vi "rqcBob KeyNET Send Data U32.vi"(8 "error in":errorcluster, 10 "Data":u32[](array[numeric]), 11 "rqcBob KeyNET in":T1) -> (0 "error out":errorcluster, 3 "rqcBob KeyNET out":T1)   [LabVIEW 2016]
uses:
  Custom Controls/rqcBob KeyNET control.ctl
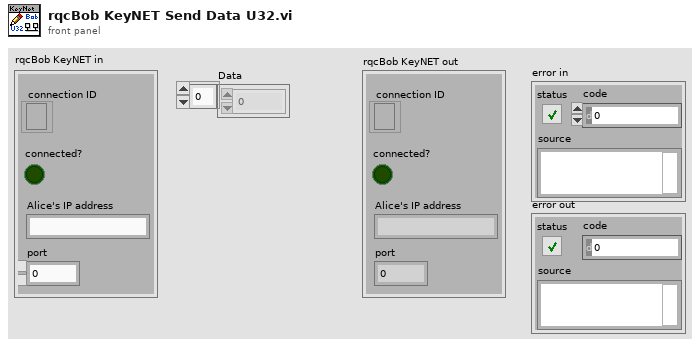
[diagram p1: front panel]
types:
  T1 = typedef "rqcBob KeyNET control.ctl" = cluster{"connection ID":refnum<k5>, "connected?":bool, "Alice's IP address":string, "port":u16}
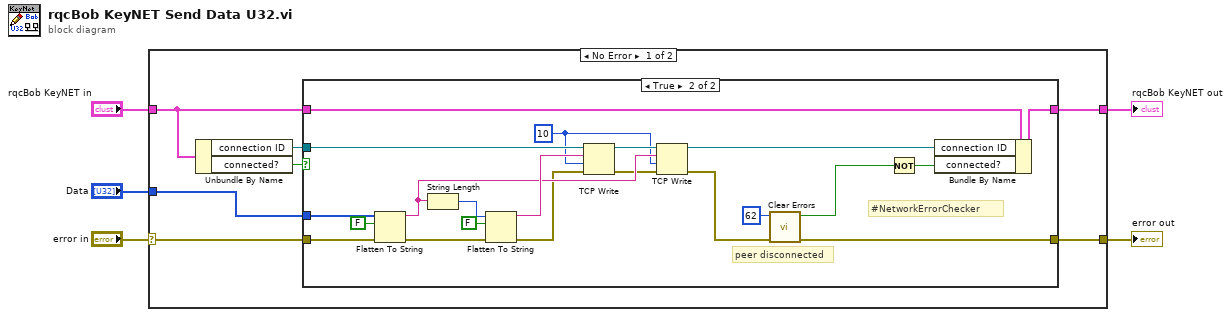
[diagram p0: block diagram]
diagram:
  n1 = case shown="No Error" "error in" {
    selector: "error in" -> [w9 w37]
    tunnel: "rqcBob KeyNET in" -> [w7 w36]
    tunnel: [w8 w37] -> w3
    tunnel: [w6 w36] -> w2
    tunnel: "Data" -> [w10 _]
    frame No Error {
      n2 = Unbundle By Name(w7) -> ("connection ID"=w11:refnum<k5>, "connected?"=w12:bool)
      n3 = case shown="True" w12 {
        tunnel: w11 -> [_ w35]
        tunnel: w10 -> [_ w34]
        tunnel: w9 -> [w14 w33]
        tunnel: [w14 w19] -> w8
        tunnel: [w13 w22] -> w6
        tunnel: w7 -> [w13 w23]
        frame False {
        }
        frame True {
          w20 = 10 ("timeout ms (25000)")
          # "peer disconnected"
          # "#NetworkErrorChecker"
          n4 = Flatten To String(anything=w34, prepend array or string size? (T)=FALSE, error in (no error)=w33) -> (data string=w28:string, error out=w31:errorcluster)  [unwired: 1 in, 1 out]
          n5 = String Length(string=w28) -> (length=w30:i32)
          n6 = Flatten To String(anything=w30, prepend array or string size? (T)=FALSE, error in (no error)=w31) -> (data string=w29:string, error out=w27:errorcluster)  [unwired: 1 in, 1 out]
          n7 = TCP Write(connection ID=w35, data in=w29, error in (no error)=w27, 9:w20) -> (connection ID out=w25:refnum<k5>, error out=w26:errorcluster)  [unwired: 1 out]
          n8 = TCP Write(connection ID=w25, data in=w28, error in (no error)=w26, 9:w20) -> (connection ID out=w21:refnum<k5>, error out=w24:errorcluster)  [unwired: 1 out]
          n9 = call <vilib>:"Clear Errors.vi"("error in (no error)"=w24, "specific error code to clear (0: all)"=62) -> ("error out"=w19:errorcluster, "specific error cleared?"=w16:bool)  [unwired: 4 in]
          n10 = Not(x=w16) -> (.not. x?=w17:bool)
          n11 = Bundle By Name(cluster=w23, "connection ID"=w21, "connected?"=w17) -> (w22:T1)
        }
      }
    }
    frame Error {
    }
  }
  "error out" <- w3
  "rqcBob KeyNET out" <- w2
